vi "test_MonoSetAndGetPosition.vi"(6 "Delay between send and receive [ms]":i32=100, 7 "Test should pass":bool=TRUE, 8 "error in":errorcluster, 9 "tear down connection":bool=TRUE, 10 "set-up a connection":bool=TRUE, 11 "device selection":enum16{"monochromator", "CCD", "SCD"}(ring)) -> (0 "error out":errorcluster, 1 "log-file path":path)   [LabVIEW 2023, in "horiba.test.lvlib"]
uses:
  horiba.test.lvlib
  <vilib>/addons/_JKI Toolkits/Caraya/classes/Test/Test.lvclass
  <vilib>/addons/_JKI Toolkits/Caraya/classes/Assert/Assert.lvclass
  Classes/horiba.lvlib
  <vilib>/addons/_JKI Toolkits/Caraya/classes/Assert/Assert Not Error.vi
  <vilib>/Hampel Software Engineering/HSE Logger/hse-logger.lvlib
  Classes/Mono/Monochromator.lvclass
  Classes/GenericDevice/GenericDevice.lvclass
panel:
  # "Connector Pane"
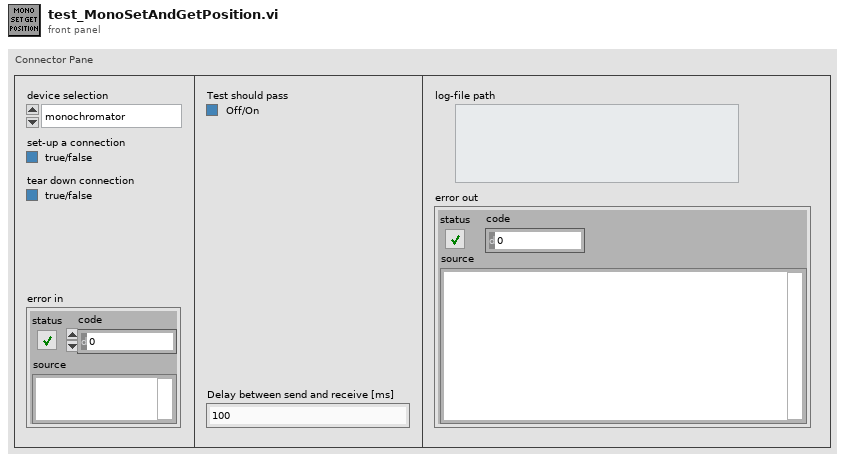
[diagram p1: front panel]
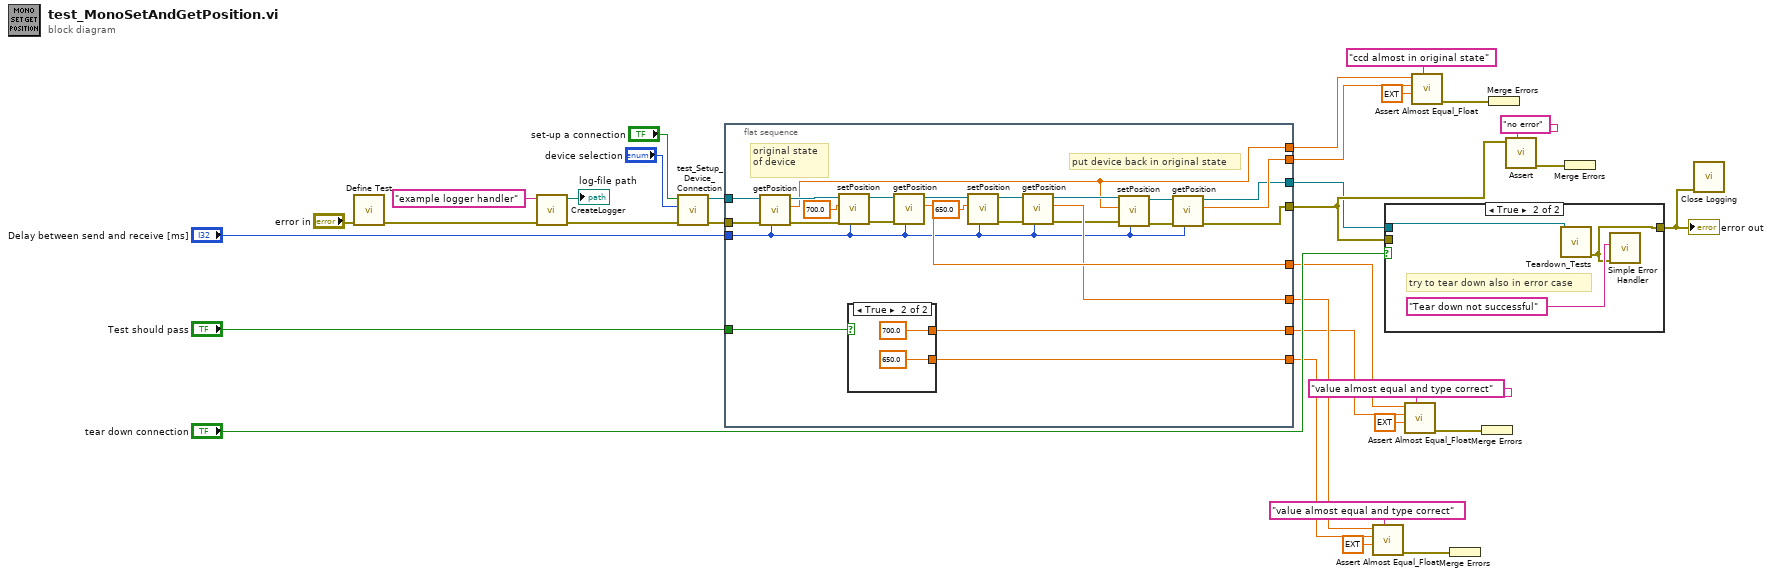
[diagram p0: block diagram]
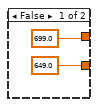
[diagram p2: hidden frame]
diagram:
  n1 = call <vilib>:"Define Test.vi"("error in (no error)"="error in") -> ("error out"=w6:errorcluster)  [unwired: 9 in, 1 out]
  n2 = call "CreateLogger.vi"("error in (no error)"=w6, "Handler Name"="example logger handler") -> ("error out"=w5:errorcluster, "log-file path"=→"log-file path":path)  [unwired: 8 in]
  n3 = call "test_Setup_Device_Connection.vi"("error in (no error)"=w5, "device selection"="device selection", "set-up a connection"="set-up a connection") -> ("error out"=w11:errorcluster, "Monochromator out"=w9:refnum<class "Monochromator.lvclass">)  [unwired: 5 in, 2 out]
  n4 = flat-sequence {
    tunnel: w11 -> [w53]
    tunnel: w9 -> [w54]
    tunnel: [w34] -> w23
    tunnel: "Test should pass" -> [w57]
    tunnel: [w35] -> w22
    tunnel: [w42] -> w21
    tunnel: [w56] -> w20
    tunnel: [w47] -> w19
    tunnel: [w55] -> w18
    tunnel: [w37] -> w15
    tunnel: [w36] -> w14
    tunnel: "Delay between send and receive [ms]" -> [w33]
    frame #0 {
      # "put device back in original state"
      # "original state of device"
      n5 = call "getPosition.vi"("Delay between send and receive [ms]"=w33, "error in (no error)"=w53, "Monochromator in"=w54) -> ("error out"=w51:errorcluster, "wavelength"=w37:dbl, "Monochromator out"=w52:refnum<class "Monochromator.lvclass">)  [unwired: 6 in]
      n6 = call "setPosition.vi"("Delay between send and receive [ms]"=w33, "error in (no error)"=w51, "wavelength"=700.0 ("exposure time [ms]"), "Monochromator in"=w52) -> ("error out"=w49:errorcluster, "Monochromator out"=w48:refnum<class "Monochromator.lvclass">)  [unwired: 4 in, 2 out]
      n7 = case shown="True" w57 {
        tunnel: [649.0 ("exposure time [ms]") 650.0 ("exposure time [ms]")] -> w56
        tunnel: [699.0 ("exposure time [ms]") 700.0 ("exposure time [ms]")] -> w55
        frame False {
        }
        frame True {
        }
      }
      n8 = call "getPosition.vi"("Delay between send and receive [ms]"=w33, "error in (no error)"=w49, "Monochromator in"=w48) -> ("wavelength"=w47:dbl, "Monochromator out"=w44:refnum<class "Monochromator.lvclass">)  [unwired: 6 in, 1 out]
      n9 = call "setPosition.vi"("Delay between send and receive [ms]"=w33, "wavelength"=650.0 ("exposure time [ms]"), "Monochromator in"=w44) -> ("error out"=w46:errorcluster, "Monochromator out"=w45:refnum<class "Monochromator.lvclass">)  [unwired: 5 in, 2 out]
      n10 = call "getPosition.vi"("Delay between send and receive [ms]"=w33, "error in (no error)"=w46, "Monochromator in"=w45) -> ("error out"=w39:errorcluster, "wavelength"=w42:dbl, "Monochromator out"=w40:refnum<class "Monochromator.lvclass">)  [unwired: 6 in]
      n11 = call "setPosition.vi"("Delay between send and receive [ms]"=w33, "error in (no error)"=w39, "wavelength"=w37, "Monochromator in"=w40) -> ("error out"=w41:errorcluster, "Monochromator out"=w38:refnum<class "Monochromator.lvclass">)  [unwired: 4 in, 2 out]
      n12 = call "getPosition.vi"("Delay between send and receive [ms]"=w33, "error in (no error)"=w41, "Monochromator in"=w38) -> ("error out"=w34:errorcluster, "wavelength"=w36:dbl, "Monochromator out"=w35:refnum<class "Monochromator.lvclass">)  [unwired: 6 in]
    }
  }
  n13 = call <vilib>:"Assert Almost Equal_Float.vi"("Label"="value almost equal and type correct" ("Label (VI Title)"), "Tolerance"=ext 0.1, "Y"=w20, "X"=w21) -> ("error out"=w31:errorcluster)  [unwired: 6 in, 1 out]
  n14 = case shown="True" "tear down connection" {
    tunnel: w22 -> [_ w64]
    tunnel: [w62 w63] -> w4
    tunnel: w23 -> [w62 _]
    frame False {
    }
    frame True {
      # "try to tear down also in error case"
      n15 = call "Teardown_Tests.vi"("horiba.lvlib:GenericDevice"=w64) -> ("error out"=w63:errorcluster)  [unwired: 9 in, 1 out]
      n16 = call <vilib>:"Simple Error Handler.vi"("error source (\" \")"="Tear down not successful" ("error source (\" \")"), "error in (no error)"=w63) -> ()  [unwired: 3 in, 5 out]
    }
  }
  "error out" <- w4
  n17 = call <vilib>:"Assert Almost Equal_Float.vi"("Label"="value almost equal and type correct" ("Label (VI Title)"), "Tolerance"=ext 0.1, "Y"=w18, "X"=w19) -> ("error out"=w30:errorcluster)  [unwired: 6 in, 1 out]
  n18 = call <vilib>:"Assert Almost Equal_Float.vi"("Label"="ccd almost in original state" ("Label (VI Title)"), "Tolerance"=ext 0.1, "Y"=w14, "X"=w15) -> ("error out"=w17:errorcluster)  [unwired: 6 in, 1 out]
  n19 = Merge Errors(w31) -> ()  [unwired: 1 out]
  n20 = Merge Errors(w30) -> ()  [unwired: 1 out]
  n21 = Merge Errors(w17) -> ()  [unwired: 1 out]
  n22 = call-poly <vilib>:"Assert.vi"("Label"="no error" ("Label (VI Title)"), "Not Error?"=w23) -> ("error out"=w25:errorcluster)  [unwired: 8 in, 1 out]
  n23 = Merge Errors(w25) -> ()  [unwired: 1 out]
  n24 = call <vilib>:"Close Logging.vi"("error in"=w4) -> ()  [unwired: 10 in, 1 out]
